vi "Init GPS.vi"() -> (3 "GPS-Compass Queue Cluster":T1)   [LabVIEW 2013]
uses:
  Data/TypeDefs/GPS-Compass Queue Cluster.ctl
  Data/TypeDefs/GPS Sensor Status.ctl
  Data/TypeDefs/UTM Location.ctl
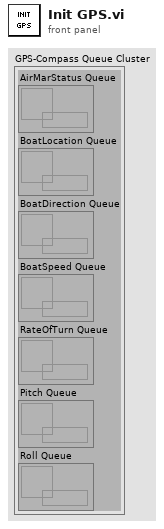
[diagram p1: front panel]
types:
  T1 = typedef "GPS-Compass Queue Cluster.ctl" = cluster{"AirMarStatus Queue":refnum<queue>, "BoatLocation Queue":refnum<queue>, "BoatDirection Queue":refnum<queue>, "BoatSpeed Queue":refnum<queue>, "RateOfTurn Queue":refnum<queue>, "Pitch Queue":refnum<queue>, "Roll Queue":refnum<queue>}
  T2 = typedef "UTM Location.ctl" = cluster{"UTM Zone":dbl, "Hemisphere":enum16{"North", "South"}, "East":dbl, "North":dbl}
  T3 = typedef "GPS Sensor Status.ctl" = cluster{"Sensor Connected":bool, "Sensor OK":bool, "GPS Lock":bool, "Sensor Initialized":bool}
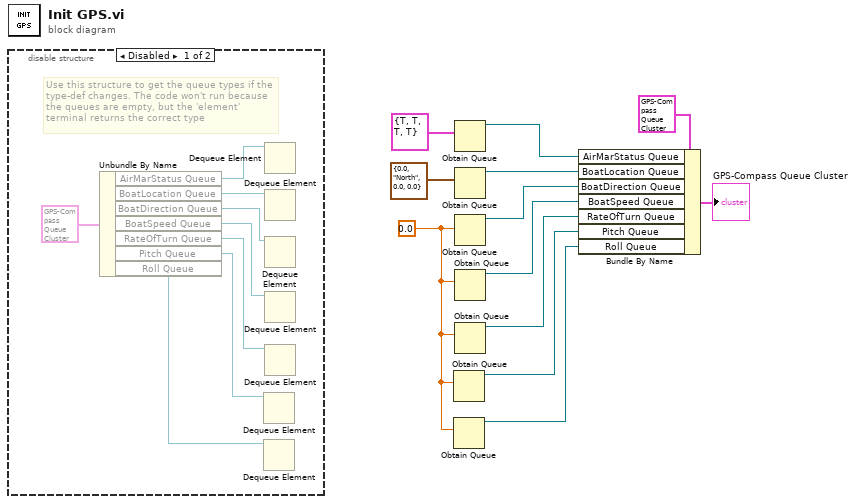
[diagram p0: block diagram]
diagram:
  w1 = 0.0 ("element")
  n1 = disable-structure shown="Disabled" {
    frame Disabled {
      # "Use this structure to get the queue types if the type-def changes. The code won't run because the queues are empty, but the 'element' terminal returns the correct type"
      n2 = Unbundle By Name(T1 {"AirMarStatus Queue"=refnum, "BoatLocation Queue"=refnum, "BoatDirection Queue"=refnum, "BoatSpeed Queue"=refnum, "RateOfTurn Queue"=refnum, "Pitch Queue"=refnum, "Roll Queue"=refnum}) -> ("AirMarStatus Queue"=w15:refnum<queue>, "BoatLocation Queue"=w16:refnum<queue>, "BoatDirection Queue"=w14:refnum<queue>, "BoatSpeed Queue"=w17:refnum<queue>, "RateOfTurn Queue"=w18:refnum<queue>, "Pitch Queue"=w19:refnum<queue>, "Roll Queue"=w20:refnum<queue>)
      n3 = Dequeue Element(queue=w19) -> ()  [unwired: 2 in, 4 out]
      n4 = Dequeue Element(queue=w20) -> ()  [unwired: 2 in, 4 out]
      n5 = Dequeue Element(queue=w15) -> ()  [unwired: 2 in, 4 out]
      n6 = Dequeue Element(queue=w16) -> ()  [unwired: 2 in, 4 out]
      n7 = Dequeue Element(queue=w14) -> ()  [unwired: 2 in, 4 out]
      n8 = Dequeue Element(queue=w17) -> ()  [unwired: 2 in, 4 out]
      n9 = Dequeue Element(queue=w18) -> ()  [unwired: 2 in, 4 out]
    }
    frame Enabled {
    }
  }
  n10 = Obtain Queue ("AirmarGPS-Compass Queue")(element data type=w1) -> (queue out=w10:refnum<queue>)  [unwired: 4 in, 2 out]
  n11 = Obtain Queue ("AirmarGPS-Compass Queue")(element data type=w1) -> (queue out=w11:refnum<queue>)  [unwired: 4 in, 2 out]
  n12 = Obtain Queue ("AirmarGPS-Compass Queue")(element data type=T3 {"Sensor Connected"=TRUE, "Sensor OK"=TRUE, "GPS Lock"=TRUE, "Sensor Initialized"=TRUE} ("element")) -> (queue out=w5:refnum<queue>)  [unwired: 4 in, 2 out]
  n13 = Obtain Queue ("AirmarGPS-Compass Queue")(element data type=T2 {"UTM Zone"=0.0, "Hemisphere"=enum."North", "East"=0.0, "North"=0.0} ("element")) -> (queue out=w6:refnum<queue>)  [unwired: 4 in, 2 out]
  n14 = Obtain Queue ("AirmarGPS-Compass Queue")(element data type=w1) -> (queue out=w7:refnum<queue>)  [unwired: 4 in, 2 out]
  n15 = Obtain Queue ("AirmarGPS-Compass Queue")(element data type=w1) -> (queue out=w9:refnum<queue>)  [unwired: 4 in, 2 out]
  n16 = Obtain Queue ("AirmarGPS-Compass Queue")(element data type=w1) -> (queue out=w8:refnum<queue>)  [unwired: 4 in, 2 out]
  n17 = Bundle By Name(cluster=T1 {"AirMarStatus Queue"=refnum, "BoatLocation Queue"=refnum, "BoatDirection Queue"=refnum, "BoatSpeed Queue"=refnum, "RateOfTurn Queue"=refnum, "Pitch Queue"=refnum, "Roll Queue"=refnum}, "AirMarStatus Queue"=w5, "BoatLocation Queue"=w6, "BoatDirection Queue"=w7, "BoatSpeed Queue"=w9, "RateOfTurn Queue"=w8, "Pitch Queue"=w10, "Roll Queue"=w11) -> (→"GPS-Compass Queue Cluster":T1)
